vi "Obtain.vi"(7 "max queue size (-1, unlimited)":i32=-1, 8 "error in (no error)":errorcluster, 9 "create if not found? (T)":bool=TRUE, 11 "name (unnamed)":string) -> (0 "error out":errorcluster, 1 "created new?":bool, 3 "queue out":refnum<queue>)   [LabVIEW 2012, in "Command Queue.lvlib"]
uses:
  <vilib>/CommandQueue/Command Queue.lvlib
  <vilib>/CommandQueue/Command.ctl
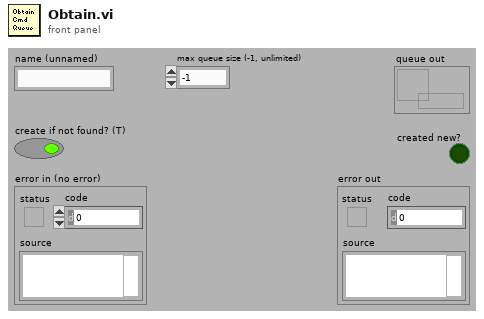
[diagram p1: front panel]
types:
  T1 = typedef "Command Queue.lvlib/Command.ctl" = cluster{"command":string, "data":variant}
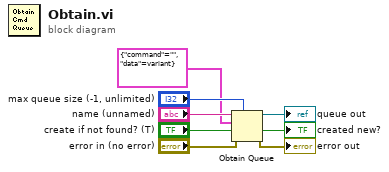
[diagram p0: block diagram]
diagram:
  n1 = Obtain Queue(max queue size (-1, unlimited)="max queue size (-1, unlimited)", name (unnamed)="name (unnamed)", element data type=T1 {"command"="", "data"=variant} ("command queue element"), create if not found? (T)="create if not found? (T)", error in (no error)="error in (no error)") -> (queue out=→"queue out":refnum<queue>, created new?=→"created new?":bool, error out=→"error out":errorcluster)
